vi "Receiver_labview_pulses.vi"() -> ()   [LabVIEW 2013]
uses:
  <vilib>/Analysis/2dsp.llb/1D Convolution (CDB).vi
  <vilib>/Analysis/2dsp.llb/Upsample (CDB).vi
  <vilib>/imath/engines/lvmath2/RunTimeEngine/ErrorHandling/NIMS_Finalize Error.vi
  <vilib>/imath/engines/lvmath2/RunTimeEngine/NodeEndStatement/NIMS_NodeEndStatement_Output.vi
  <instcachedir>/0/NIMS_NodeEndStatement_Output_53EC0D466D134D7ABD903AC30B43404B.lvgen/NIMS_NodeEndStatement_Output_53EC0D466D134D7ABD903AC30B43404B_004.vi
  <vilib>/imath/engines/lvmath2/RunTimeEngine/BuiltInFunctions/randint/NIMS_randint(1,I32,RV).vi
  <vilib>/imath/engines/lvmath2/RunTimeEngine/ErrorHandling/NIMS_Create Error From Enums.vi
  <vilib>/Analysis/NI_AALPro.lvlib
panel:
  in  "Sampling frequency 2":dbl=30000000.0
  out "After Matched Filtering":dbl[](graph)
  in  "Symbol frequency 2":dbl
  in  "Sampling frequency":dbl=30000000.0
  out "number of symbols (per block)":dbl
  out "Baseband Signal":dbl[](graph)
  out "Root Raise Cosine Pulse":dbl[](graph)
  out "Constellation (16-QAM)":cdb[](graph)
  in  "Symbol frequency":dbl
  in  "number of bits (per block)":dbl
  out "First Start":dbl(graph)
  out "Waveform Chart 2":dbl(graph)
  in  "stop":bool
  out "Symbols 1":cdb[](graph)
  out "Symbols 2":cdb[](graph)
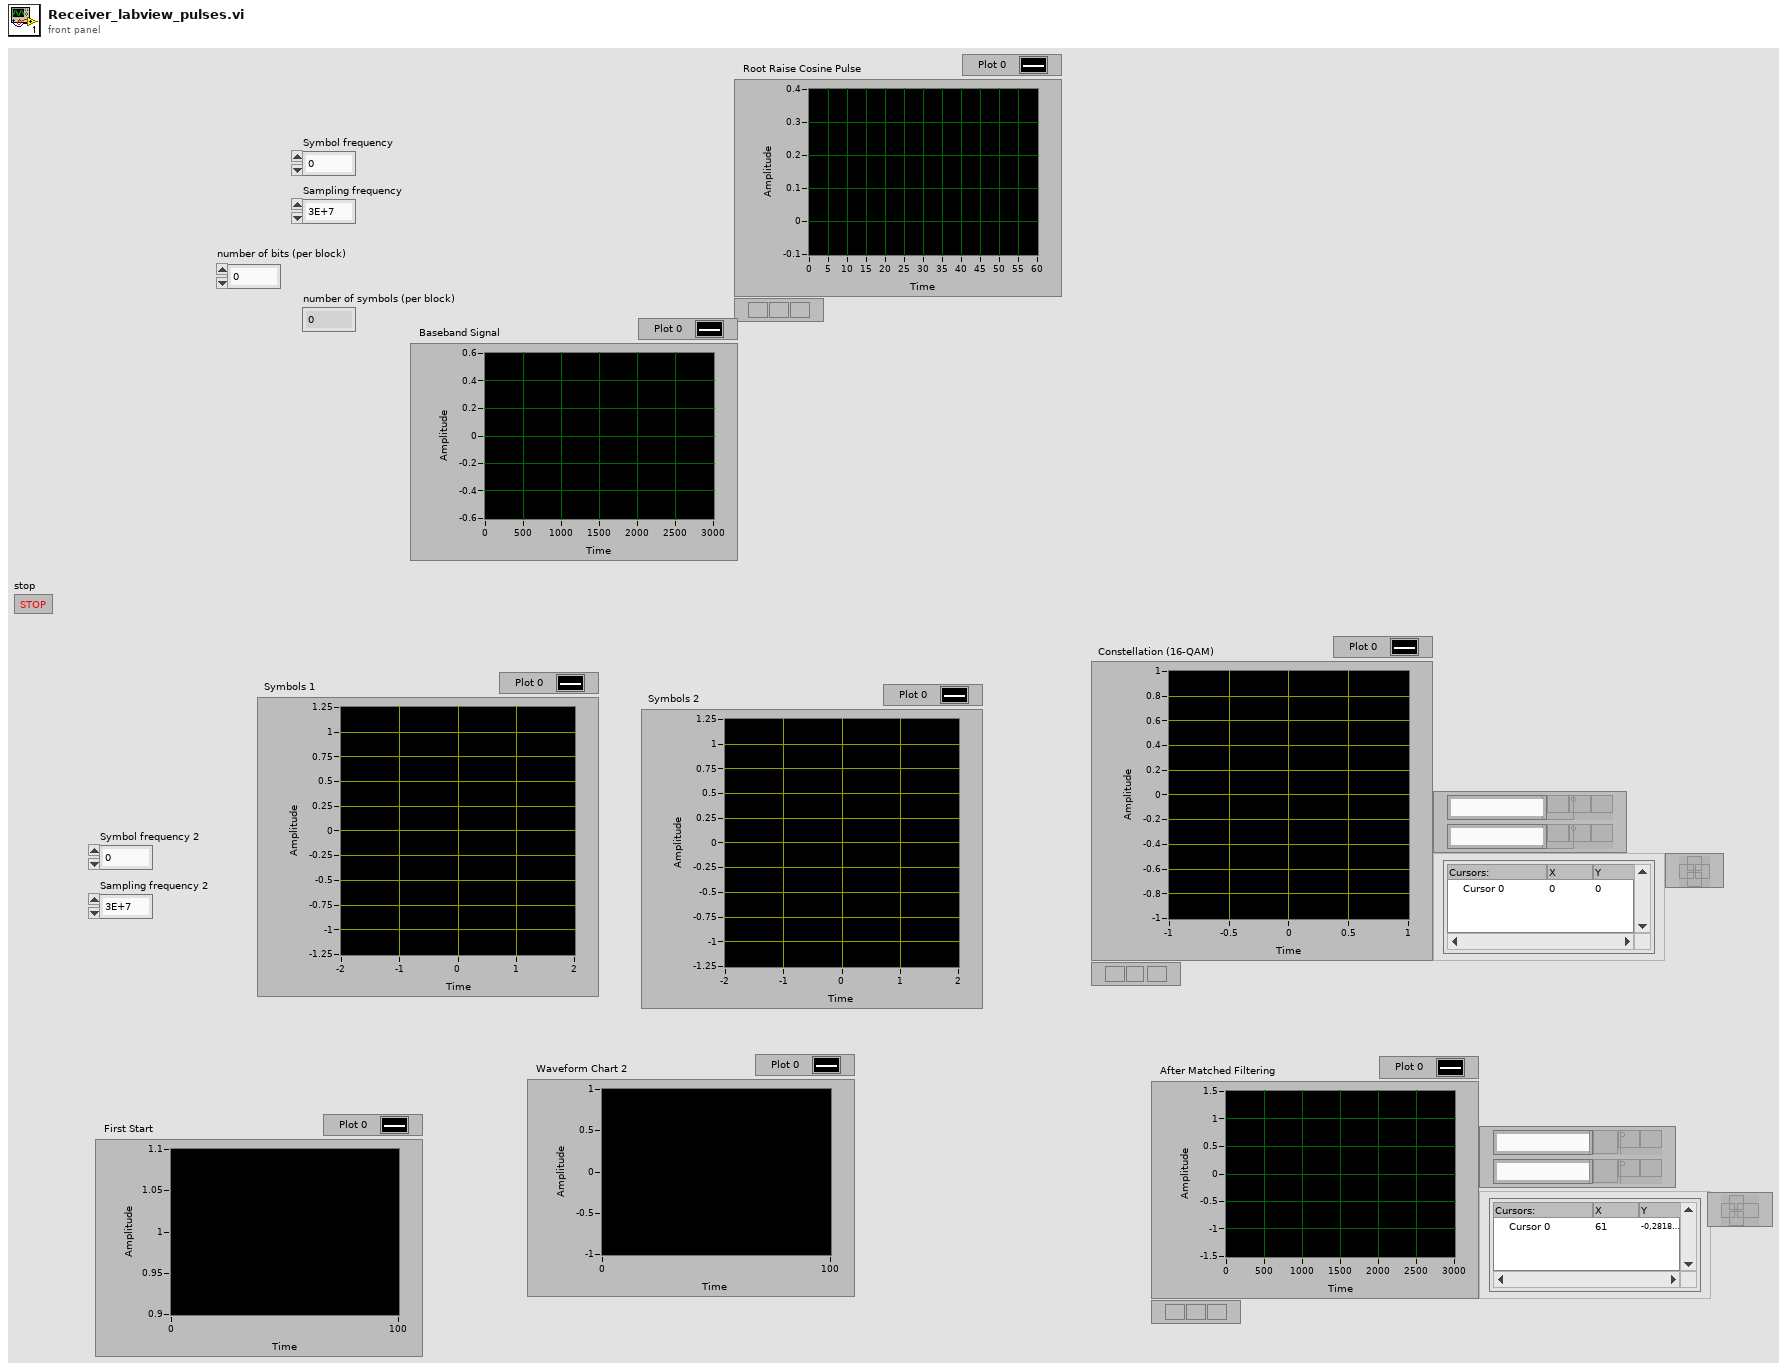
[diagram p1: front panel]
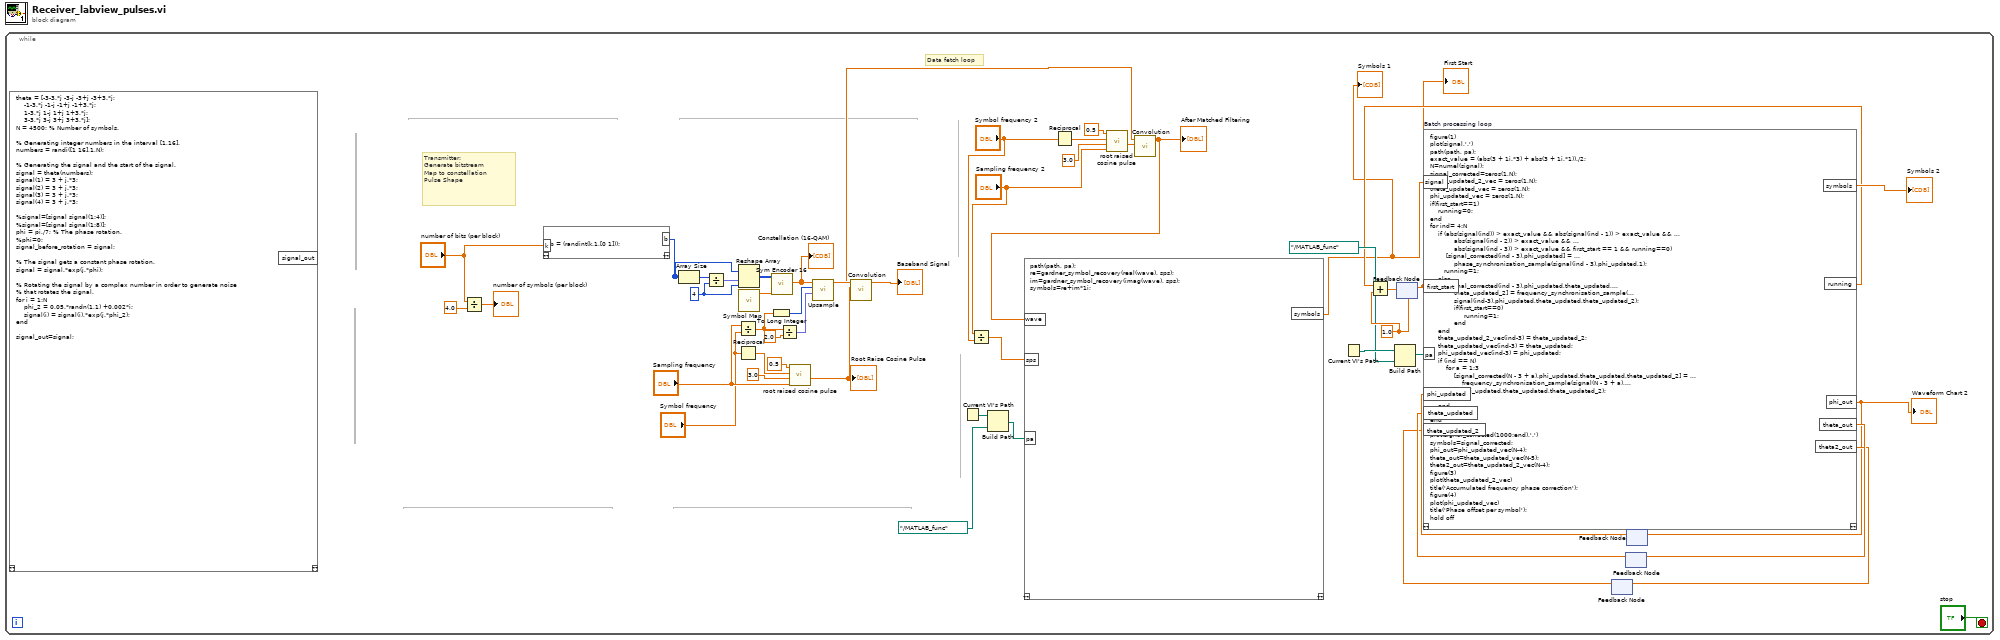
[diagram p0: block diagram]
diagram:
  n1 = while {
    stop <- "stop" stop-if-true
    w19 = 4 ("dimension size")
    w43 = 1.0
    # "Transmitter:\nGenerate bitstream\nMap to constellation\nPulse Shape"
    # "Data fetch loop"
    n2 = script code="theta = [-3-3.*j -3-j -3+j -3+3.*j;\n    -1-3.*j -1-j -1+j -1+3.*j;\n    1-3.*j 1-j 1+j 1+3.*j;\n    3-3.*j 3-j 3+j 3+3.*j];\nN = 4500; % Number of symbols.\n\n% Generating integer numbers in the interval [1,16].\nnumbers = randi([1 16],1,N);\n\n% Generating the signal and the start of the signal.\nsignal = theta(numbers);\nsignal(1) = 3 + j.*3;\nsignal(2) = 3 + j.*3;\nsignal(3) = 3 + j.*3;\nsignal(4) = 3 + j.*3;\n\n%signal=[signal signal(1:4)];\n%signal=[signal signal(1:8)];\nphi = pi./7; % The phase rotation.\n%phi=0;\nsignal_before_rotation = signal;\n\n% The signal gets a constant phase rotation.\nsignal = signal.*exp(j.*phi);\n\n% Rotating the signal by a complex number in order to generate noise\n% that rotates the signal.\nfor i = 1:N\n    phi_2 = 0.05.*randn(1,1) +0.002*i;\n    signal(i) = signal(i).*exp(j.*phi_2);\nend\n\nsignal_out=signal;"() -> ()  [unwired: 1 in, 2 out]
    n3 = Divide(x="number of bits (per block)", y=4.0) -> (x/y=→"number of symbols (per block)":dbl)
    n4 = mathscript code="b = (randint(k,1,[0 1]));"("k"="number of bits (per block)") -> ("b"=w14:i32[])  [unwired: 1 in, 1 out]
    n5 = Array Size(array=w14) -> (size(s)=w17:i32)
    n6 = Divide(x=w17, y=w19) -> (x/y=w18:fxp<+,27,27>)
    n7 = Divide(x="Sampling frequency", y="Symbol frequency") -> (x/y=w26:dbl)
    n8 = Reciprocal(x="Symbol frequency") -> (1/x=w29:dbl)
    n9 = Reshape Array(w14, w18, w19) -> (w21:i32[][])
    n10 = call "Symbol Map.vi"() -> ("symbol_map"=w20:cdb[])  [unwired: 11 in]
    n11 = To Long Integer(number=w26) -> (32bit integer=w27:i32)
    n12 = call "Sym Encoder 16.vi"("symbol_map"=w20, "b"=w21) -> ("a"=w22:cdb[])  [unwired: 9 in]
    "Constellation (16-QAM)" <- w22
    n13 = Divide(x=w26, y=2.0) -> (x/y=w34:fxp<+,32,32>)
    n14 = call "root raised cosine pulse.vi"("fs"="Sampling frequency", "span"=3.0, "tau"=w29, "a"=0.5) -> ("y"=w24:cdb[])  [unwired: 6 in, 1 out]
    "Root Raise Cosine Pulse" <- w24
    n15 = call-poly <vilib>:"Upsample.vi"("leading zeros"=w34, "upsampling factor"=w27, "X"=w22) -> ("Upsampled Array"=w23:cdb[])  [unwired: 7 in, 1 out]
    n16 = call-poly <vilib>:"Convolution.vi"("Y"=w24, "X"=w23) -> ("X * Y"=w9:cdb[])  [unwired: 8 in, 1 out]
    "Baseband Signal" <- w9
    n17 = Current VI's Path() -> (path=w4:path)
    n18 = Divide(x="Sampling frequency 2", y="Symbol frequency 2") -> (x/y=w8:dbl)
    n19 = Build Path(base path=w4, name or relative path=path "../MATLAB_func") -> (appended path=w5:path)
    n20 = Reciprocal(x="Symbol frequency 2") -> (1/x=w13:dbl)
    n21 = call "root raised cosine pulse.vi"("fs"="Sampling frequency 2", "span"=3.0, "tau"=w13, "a"=0.5) -> ("y"=w12:cdb[])  [unwired: 6 in, 1 out]
    n22 = call-poly <vilib>:"Convolution.vi"("Y"=w12, "X"=w9) -> ("X * Y"=w2:cdb[])  [unwired: 8 in, 1 out]
    "After Matched Filtering" <- w2
    n23 = script code="path(path, pa);\nre=gardner_symbol_recovery(real(wave), sps);\nim=gardner_symbol_recovery(imag(wave), sps);\nsymbols=re+im*1i;"("wave"=w2, "sps"=w8, "pa"=w5) -> ("symbols"=w1:cdb[])  [unwired: 1 in, 1 out]
    "Symbols 1" <- w1
    n24 = Current VI's Path() -> (path=w40:path)
    n25 = Build Path(base path=w40, name or relative path=path "../MATLAB_func") -> (appended path=w41:path)
    n26 = feedback #1(w43) -> (w35:dbl)
    "First Start" <- w35
    n27 = feedback #2() -> (w45:dbl)  [unwired: 1 in]
    n28 = feedback #3() -> (w47:dbl)  [unwired: 1 in]
    n29 = feedback #4() -> (w49:dbl)  [unwired: 1 in]
    n30 = script code="figure(1)\nplot(signal,'.')\npath(path, pa);\nexact_value = (abs(3 + 1i.*3) + abs(3 + 1i.*1))./2;\nN=numel(signal);\nsignal_corrected=zeros(1,N);\ntheta_updated_2_vec = zeros(1,N);\ntheta_updated_vec = zeros(1,N);\nphi_updated_vec = zeros(1,N);\nif(first_start==1)\n    running=0;\nend\nfor ind= 4:N\n    if (abs(signal(ind)) > exact_value && abs(signal(ind - 1)) > exact_value && ...\n            abs(signal(ind - 2)) > exact_value && ...\n            abs(signal(ind - 3)) > exact_value && first_start == 1 && running==0)\n        [signal_corrected(ind - 3),phi_updated] = ...\n            phase_synchronisation_sample(signal(ind - 3),phi_updated,1);\n       running=1;\n    else\n        [signal_corrected(ind - 3),phi_updated,theta_updated,...\n            theta_updated_2] = frequency_synchronisation_sample(...\n            signal(ind-3),phi_updated,theta_updated,theta_updated_2);\n            if(first_start==0)\n                 running=1;\n            end\n    end\n    theta_updated_2_vec(ind-3) = theta_updated_2;\n    theta_updated_vec(ind-3) = theta_updated;\n    phi_updated_vec(ind-3) = phi_updated;\n    if (ind == N)\n        for a = 1:3\n            [signal_corrected(N - 3 + a),phi_updated,theta_updated,theta_updated_2] = ...\n                frequency_synchronisation_sample(signal(N - 3 + a),...\n                phi_updated,theta_updated,theta_updated_2);\n        end\n    end\n\nend\nfigure(2)\nplot(signal_corrected(1000:end),'.')\nsymbols=signal_corrected;\nphi_out=phi_updated_vec(N-4);\ntheta_out=theta_updated_vec(N-5);\ntheta2_out=theta_updated_2_vec(N-4);\nfigure(3)\nplot(theta_updated_2_vec)\ntitle('Accumulated frequency phase correction');\nfigure(4)\nplot(phi_updated_vec)\ntitle('Phase offset per symbol');\nhold off" "Batch processing loop"("signal"=w1, "first_start"=w35, "phi_updated"=w49, "theta_updated"=w47, "theta_updated_2"=w45, "pa"=w41) -> ("phi_out"=w36:dbl, "theta_out"=w48:dbl, "theta2_out"=w46:dbl, "symbols"=→"Symbols 2":cdb[], "running"=w37:dbl)  [unwired: 1 in, 1 out]
    "Waveform Chart 2" <- w36
    n31 = Add(x=w37, y=w43) -> (x+y=w44:dbl)
    n32 = feedback-in #1(w44) -> ()
    n33 = feedback-in #2(w46) -> ()
    n34 = feedback-in #3(w48) -> ()
    n35 = feedback-in #4(w36) -> ()
  }
